vi "Configure Laser Output.vi"(8 "error in":errorcluster, 11 "PAS in":refnum<class "PAS.lvclass">) -> (0 "error out":errorcluster, 3 "PAS out":refnum<class "PAS.lvclass">)   [LabVIEW 2014, in "PAS.lvclass"]
doc: "Configure the output for the laser. This method is implementation dependent and must be overridden by the current instance. THIS VI IS ABSTRACT."
uses:
  PAS.lvclass
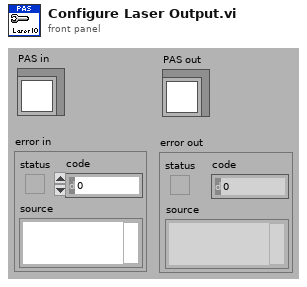
[diagram p1: front panel]
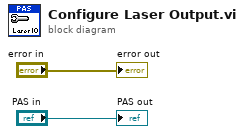
[diagram p0: block diagram]
diagram:
  "error out" <- "error in"
  "PAS out" <- "PAS in"
